vi "trace.vi"(8 "error in (no error)":errorcluster, 10 "para2":u32, 11 "para0":dbl) -> (0 "error out":errorcluster, 1 "function return":u32, 2 "para2 out":u32, 3 "para0 out":dbl)   [LabVIEW 2020, in "sqlite3.lvlib"]
uses:
  sqlite3.lvlib
  errstr.vi
  bin/sqlite3_64.dll
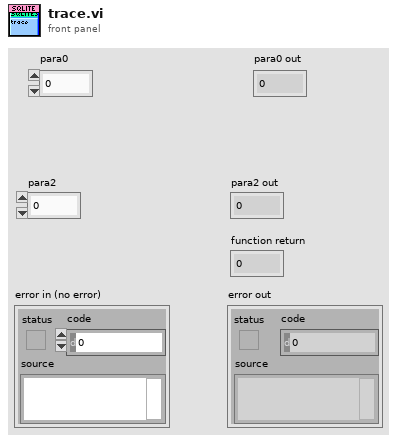
[diagram p1: front panel]
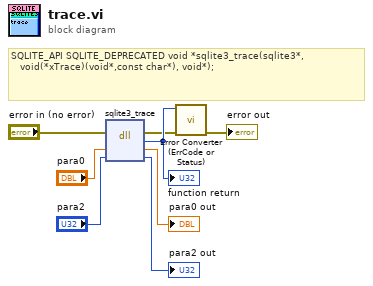
[diagram p0: block diagram]
diagram:
  # "SQLITE_API SQLITE_DEPRECATED void *sqlite3_trace(sqlite3*,\n   void(*xTrace)(void*,const char*), void*);"
  n1 = dll-call lib="C:/Users/Fred.Guo/Desktop/Database-configuration/externals/sqlite3/Source/bin/sqlite3_*.*" fn="sqlite3_trace"(error in="error in (no error)", "para0"="para0", "para2"="para2") -> (error out=w2:errorcluster, w8:u32, "para0"=→"para0 out":dbl, "para2"=→"para2 out":u32)  [unwired: 2 in, 1 out]
  "function return" <- w8
  n2 = call "Error Converter (ErrCode or Status).vi"("error in (no error)"=w2, "error code"=w8) -> ("error out"=→"error out":errorcluster)  [unwired: 9 in]
